vi "_PC_RTLoop_System_Monitor.vi"(7 "Function":enum16{"Init", "Get Data", "Close"}(ring), 8 "error in (no error)":errorcluster, 10 "Instrument Parmeter":T1) -> (0 "error out":errorcluster)   [LabVIEW 2018]
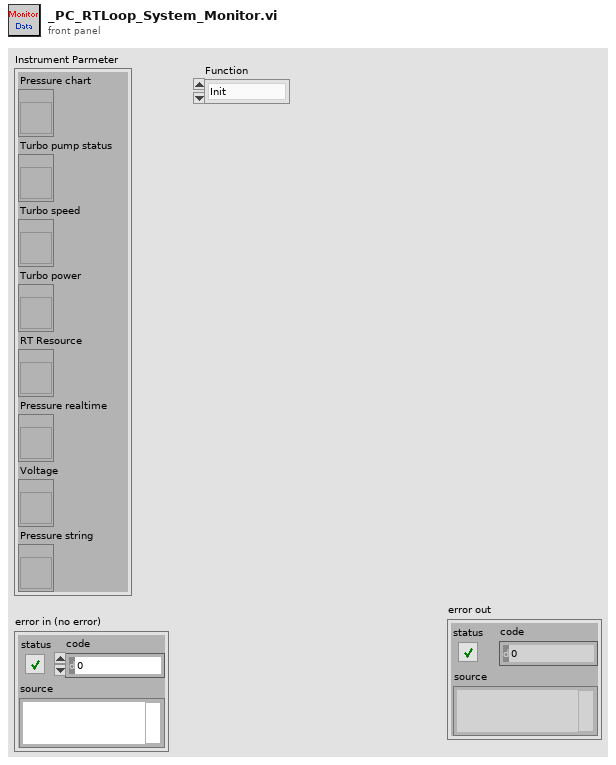
[diagram p1: front panel]
types:
  T1 = cluster{"Pressure chart":refnum<vi>, "Turbo pump status":refnum<vi>, "Turbo speed":refnum<vi>, "Turbo power":refnum<vi>, "RT Resource":refnum<vi>, "Pressure realtime":refnum<vi>, "Voltage":refnum<vi>, "Pressure string":refnum<vi>}
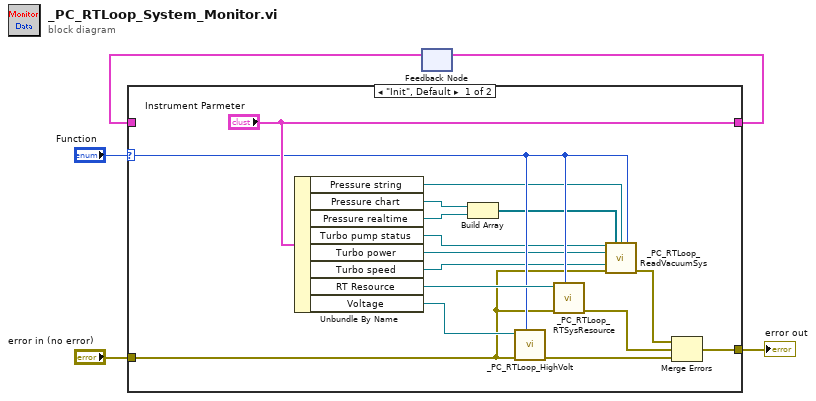
[diagram p0: block diagram]
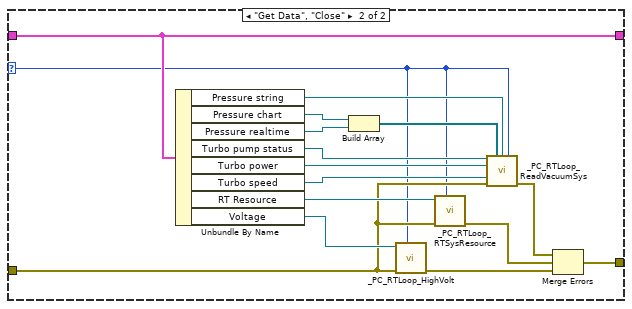
[diagram p2: hidden frame]
diagram:
  n1 = feedback #1() -> (w4:T1)  [unwired: 1 in]
  n2 = case shown="\"Init\", Default" "Function" {
    selector: "Function" -> [w18 w22]
    tunnel: w4 -> [_ w25]
    tunnel: ["Instrument Parmeter" w25] -> w5
    tunnel: "error in (no error)" -> [w10 w24]
    tunnel: [w6 w23] -> w2
    frame "Init", Default {
      n3 = Unbundle By Name("Instrument Parmeter") -> ("Pressure string"=w17:refnum<vi>, "Pressure chart"=w16:refnum<vi>, "Pressure realtime"=w15:refnum<vi>, "Turbo pump status"=w11:refnum<vi>, "Turbo power"=w13:refnum<vi>, "Turbo speed"=w12:refnum<vi>, "RT Resource"=w21:refnum<vi>, "Voltage"=w19:refnum<vi>)
      n4 = Build Array(w16, w15) -> (w14:refnum<vi>[])
      n5 = call "_PC_RTLoop_HighVolt.vi"("Function"=w18, "error in (no error)"=w10, "Voltage"=w19) -> ("error out"=w7:errorcluster)  [unwired: 8 in]
      n6 = call "_PC_RTLoop_RTSysResource.vi"("Function"=w18, "error in (no error)"=w10, "RT Resource XY Graph"=w21) -> ("error out"=w8:errorcluster)  [unwired: 8 in]
      n7 = call "_PC_RTLoop_ReadVacuumSys.vi"("string for turbo pump status"=w11, "XYGraph for pressure"=w14, "String refin"=w17, "Function"=w18, "XYGraph for Turbo power"=w13, "XYGraph for Turbo speed"=w12, "error in (no error)"=w10) -> ("error out"=w9:errorcluster)  [unwired: 8 in]
      n8 = Merge Errors(w9, w8, w7) -> (w6:errorcluster)
    }
    frame "Get Data", "Close" {
      n9 = Unbundle By Name(w25) -> ("Pressure string"=w35:refnum<vi>, "Pressure chart"=w34:refnum<vi>, "Pressure realtime"=w33:refnum<vi>, "Turbo pump status"=w29:refnum<vi>, "Turbo power"=w31:refnum<vi>, "Turbo speed"=w30:refnum<vi>, "RT Resource"=w37:refnum<vi>, "Voltage"=w36:refnum<vi>)
      n10 = Build Array(w34, w33) -> (w32:refnum<vi>[])
      n11 = call "_PC_RTLoop_HighVolt.vi"("Function"=w22, "error in (no error)"=w24, "Voltage"=w36) -> ("error out"=w26:errorcluster)  [unwired: 8 in]
      n12 = call "_PC_RTLoop_RTSysResource.vi"("Function"=w22, "error in (no error)"=w24, "RT Resource XY Graph"=w37) -> ("error out"=w27:errorcluster)  [unwired: 8 in]
      n13 = call "_PC_RTLoop_ReadVacuumSys.vi"("string for turbo pump status"=w29, "XYGraph for pressure"=w32, "String refin"=w35, "Function"=w22, "XYGraph for Turbo power"=w31, "XYGraph for Turbo speed"=w30, "error in (no error)"=w24) -> ("error out"=w28:errorcluster)  [unwired: 8 in]
      n14 = Merge Errors(w28, w27, w26) -> (w23:errorcluster)
    }
  }
  "error out" <- w2
  n15 = feedback-in #1(w5) -> ()
